vi "Oscilloscope.vi"(6 "Slow Control User":string, 9 "notifier in":T4, 10 "queue in":T3) -> ()   [LabVIEW 2012]
uses:
  TypeDefs/QueueNotifier/Notifier.ctl
  TypeDefs/QueueNotifier/DataQueue.ctl
  TypeDefs/DataTypes/SystemStatus.ctl
  TypeDefs/DataTypes/StopCondition.ctl
  TypeDefs/DataTypes/AcquisitionInfo.ctl
  TypeDefs/DataTypes/OscilloscopeState.ctl
  <vilib>/Analysis/6fits.llb/Remove Outliers (Range).vi
  <vilib>/Analysis/NI_AALPro.lvlib
panel:
  in  "Acquisition Info":T1 {"Shaping Amplifier" items=["CR-200-1us", "CR-200-100ns", "", ""]; "Preamplifier" items=["CR-Z-113-1k", "CR-Z-113-5k", "CR-Z-SiPM", ""]}
  out "Acquisition Rate":dbl format="%#.1f"
  in  "Stop":bool
  in  "Trigger Level (V)":dbl=-0.02
  in  "Range (V)":dbl(ring)=2.0 items=["10"=10.0, "5"=5.0, "2"=2.0, "1"=1.0, "0.4"=0.4, "0.2"=0.2, "0.08"=0.08, "0.04"=0.04, "0.02"=0.02, "0.01"=0.01]
  in  "Offset (V)":dbl=-0.5
  out "Acquiring Now?":bool
  out "Active Run?":bool
  out "Time Elapsed (s)":dbl format="%#.1f"
  out "Waveforms Acquired":dbl
  in  "Stop Condition":T2={"Quota"=2000.0, "Duration (S)"=120, "Stop Condition"=FALSE}
  in  "Run Info":bool caption="Configure DAQ"
  out "Signal":waveform(dbl)(graph)
  in  "Measurement (Ch1)":i32(ring)=26 items=["AC RMS"=1, "Amplitude"=2, "Average"=3, "Cycle Average"=4, "Cycle Frequency"=5, "Cycle Period"=6, "Cycle RMS"=7, "DC RMS"=8, "Estimated Number of Bits"=9, "Falling Edges"=10, "Fall Overshoot"=11, "Fall Preshoot"=12, "Frequency"=13, "Fall Crossing Time"=14, "Fall Time"=15, "High"=16, "Low"=17, "Maximum"=18, "Minimum"=19, "Mid"=20, "Negative Duty"=21, "Negative Width"=22, "Positive Duty"=23, "Period"=24, "Phase"=25, "Peak to Peak"=26, "Positive Width"=27, "Rising Edges"=28, "Rise Overshoot"=29, "Rise Preshoot"=30, "Rise Crossing Time"=31, "Rise Time"=32, "Standard Deviation"=33, "Spurious Free Dynamic Range"=34, "Signal to Noise+Distortion"=35, "Signal to Noise"=36, "Total Harmonic Distortion"=37, "Time of Maximum"=38, "Time of Minimum"=39]
  in  "New Run":bool caption="Configure DAQ"
  in  "Settings":bool caption="Configure DAQ"
  in  "Acquire":bool
  out "Preliminary Histogram":cluster{"Y":dbl[], "Y":dbl[]}[](graph)
  # "Shaper Gain"
  # "Self"
  # "Fast"
  # "Solicited"
  # "Standard"
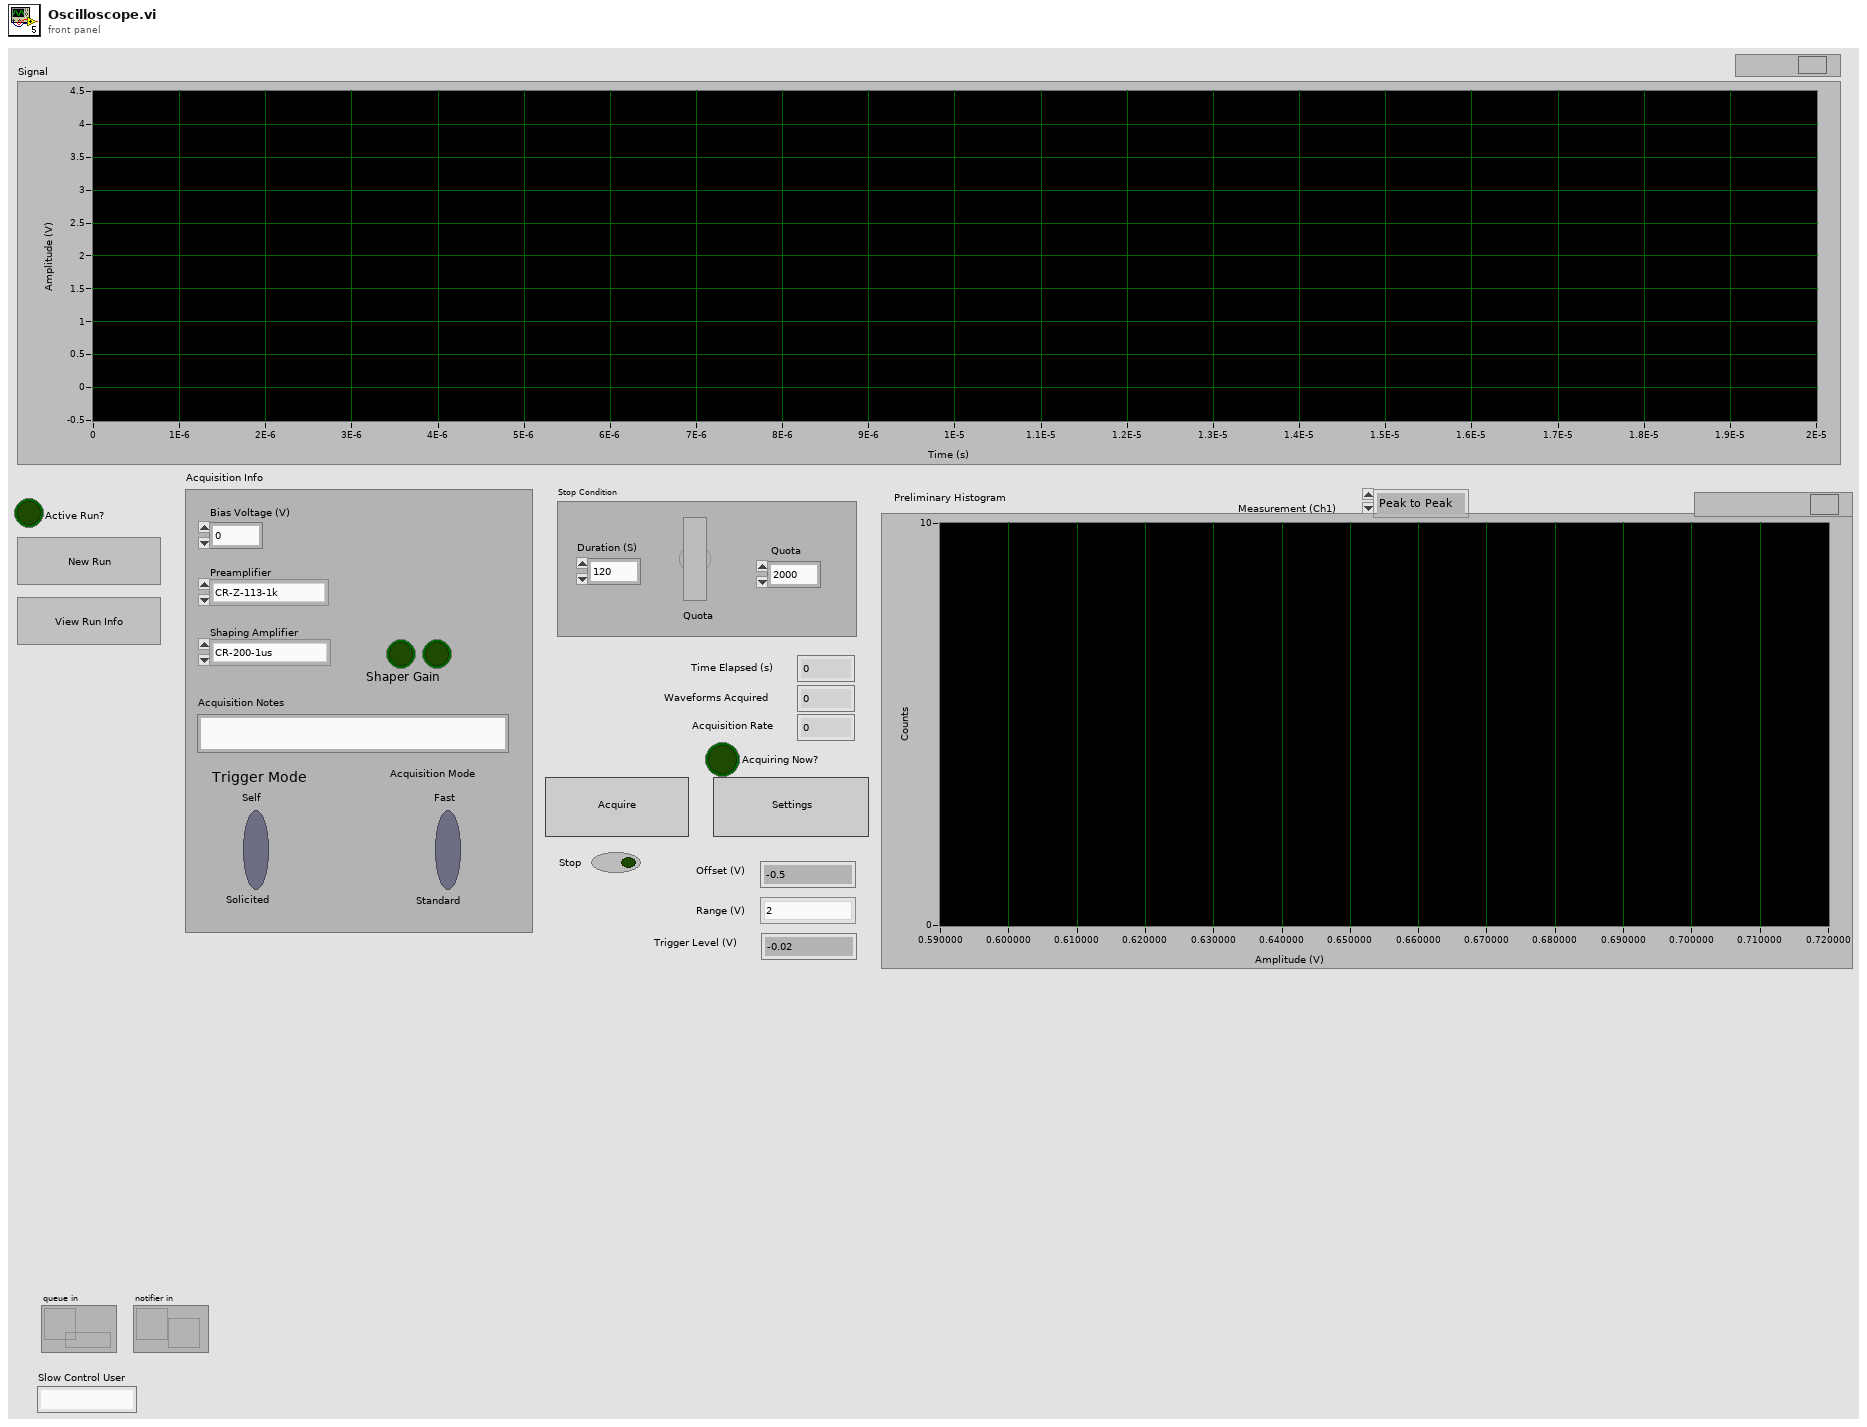
[diagram p1: front panel]
types:
  T1 = typedef "AcquisitionInfo.ctl" = cluster{"Trigger Mode":bool, "Acquisition Mode":bool, "Bias Voltage (V)":dbl, "Preamplifier":u16, "Shaping Amplifier":u16, "Acquisition Notes":string, "1":bool, "2":bool}
  T2 = typedef "StopCondition.ctl" = cluster{"Quota":dbl, "Duration (S)":u16, "Stop Condition":bool}
  T3 = typedef "DataQueue.ctl" = refnum<queue>
  T4 = typedef "Notifier.ctl" = refnum<notifier>
  T5 = typedef "OscilloscopeState.ctl" = enum16{"Acquire", "Initialize", "Waiting For Event", "New Run", "Settings", "Update UI", "ViewRunInfo", "Synchronize", "Fast Acquire"}
  T6 = typedef "Data.ctl" = cluster{"DAQ Config Data":T7, "Acquisition":T8, "Measurement":T10, "UI References":T11, "Run Info":T12, "System Status":T13, "Acquisition Info":cluster{"Trigger Mode":bool, "Acquisition Mode":bool, "Bias Voltage (V)":dbl, "Preamplifier":u16, "Shaping Amplifier":u16, "Acquisition Notes":string, "1":bool, "2":bool}}
  T7 = typedef "DAQConfig.ctl" = cluster{"Vertical":cluster{"Coupling":i32, "Offset (V)":dbl, "Range (V)":dbl, "Impedance":dbl}, "Horizontal":cluster{"Offset Time":dbl, "Sample Time (S)":dbl, "Sample Points":u32}, "Trigger\n":cluster{"Lower Level (V)":dbl, "Trigger Slope":i32, "Trigger Source":i32}, "Acquisition":cluster{"Trigger Mode":i32, "Initiate Continuously":i32, "Acquire Type":i32, "Acquire Count":i32}, "Channel":i32, "Instrument Handle":i32, "Error":errorcluster, "State":i32}
  T8 = typedef "Acquisition.ctl" = cluster{"Current":T9, "Stop Condition":T2, "Config Needed":bool}
  T9 = typedef "Current.ctl" = cluster{"Acquiring Now?":bool, "Waveforms Acquired":dbl, "Start of Acquisition":timestamp, "Acquisition Name":string}
  T10 = typedef "Measurement.ctl" = cluster{"Waveform":waveform(dbl), "Peak Heights":dbl[], "Acquisition Time":timestamp, "File Path":path, "TDMS File Handle":refnum<k34>}
  T11 = typedef "UIReferences.ctl" = cluster{"Acquire":refnum<vi>, "Configure DAQ":refnum<vi>, "Measurement (Ch1)":refnum<vi>, "Update Needed?":bool, "New Run":refnum<vi>, "Signal":refnum<vi>}
  T12 = typedef "RunInfo.ctl" = cluster{"Active Run?":bool, "Run Notes":string, "User Name":string, "Campaign ID#":string, "Run Name":string, "Start Time":timestamp, "End Time":timestamp}
  T13 = typedef "SystemStatus.ctl" = cluster{"Bias Voltage":dbl, "SiPM Temperature":dbl[], "Slow Control User":string, "LXe":dbl}
  T14 = enum8{"Enabled", "Disabled", "Disabled and Grayed Out"}
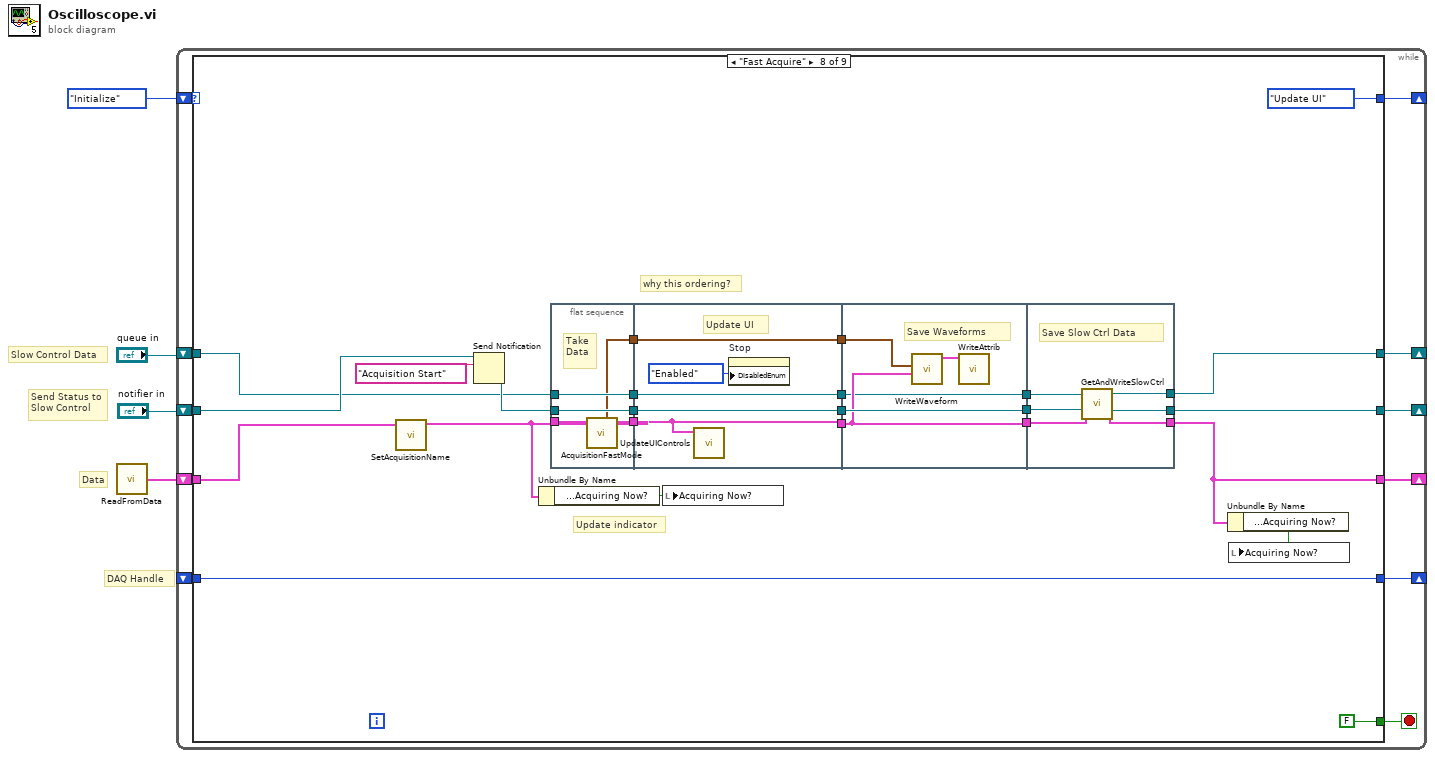
[diagram p0: block diagram]
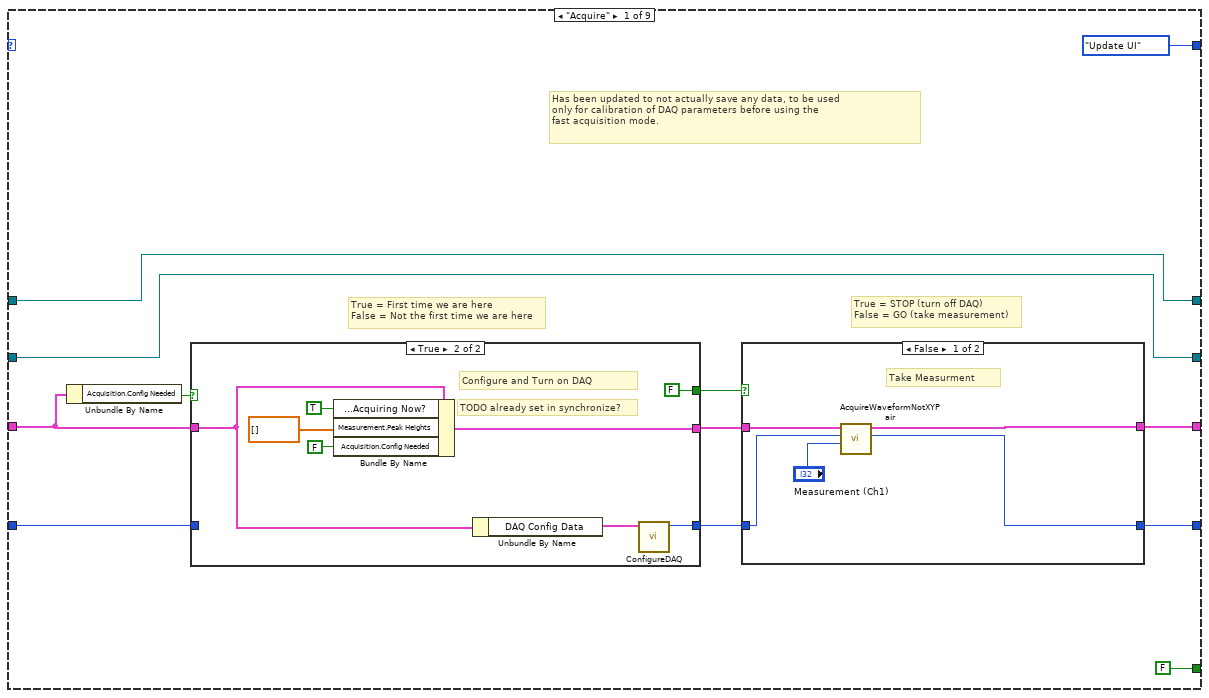
[diagram p2: hidden frame]
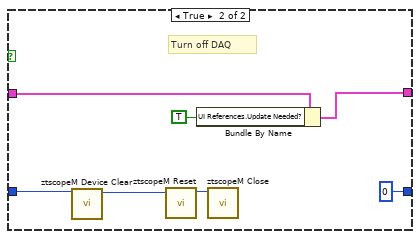
[diagram p3: hidden frame]
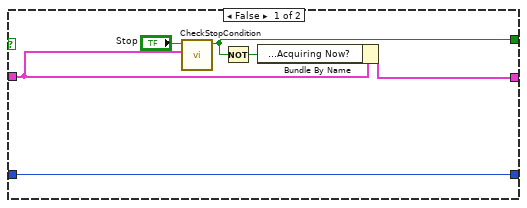
[diagram p4: hidden frame]
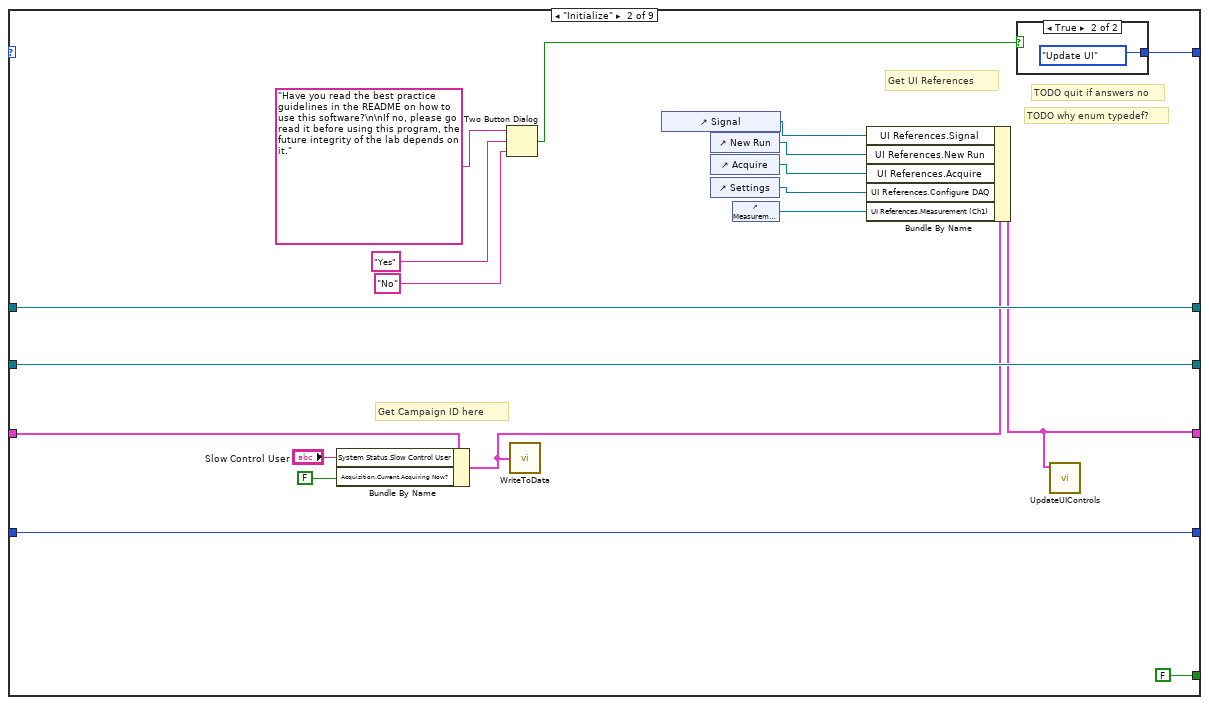
[diagram p5: hidden frame]
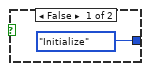
[diagram p6: hidden frame]
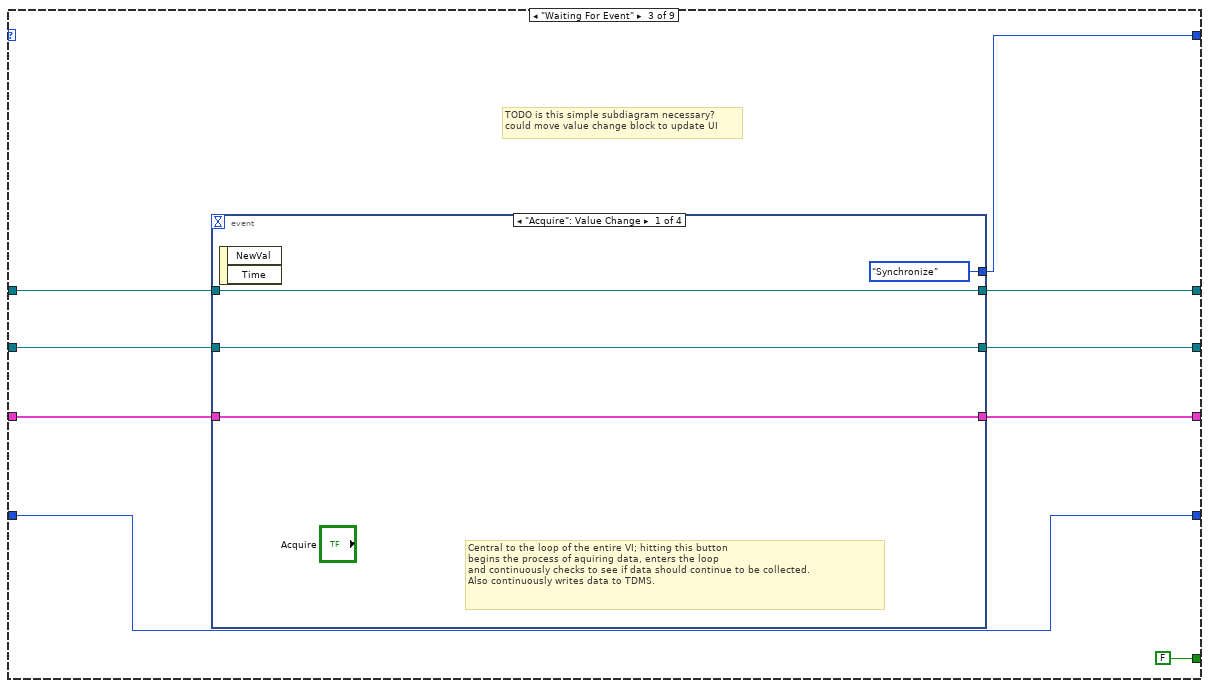
[diagram p7: hidden frame]
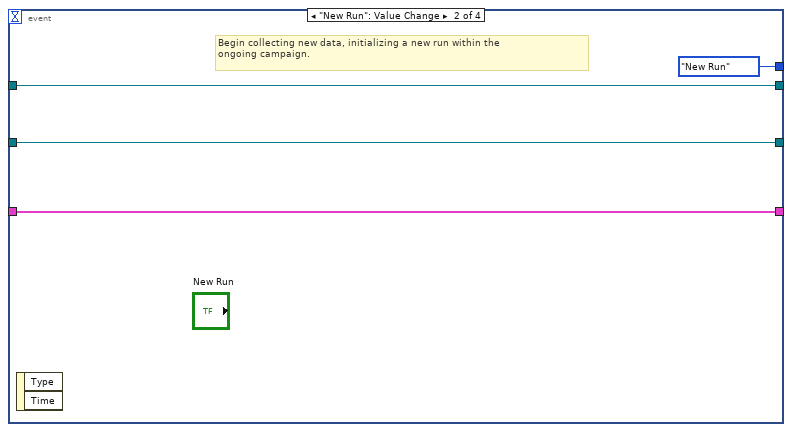
[diagram p8: hidden frame]
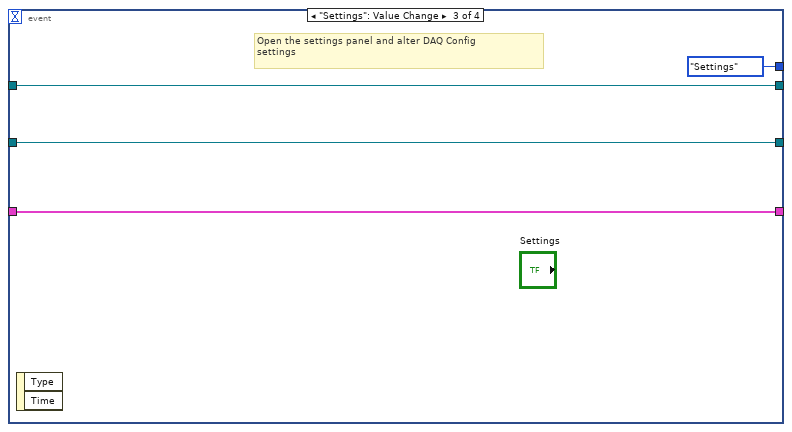
[diagram p9: hidden frame]
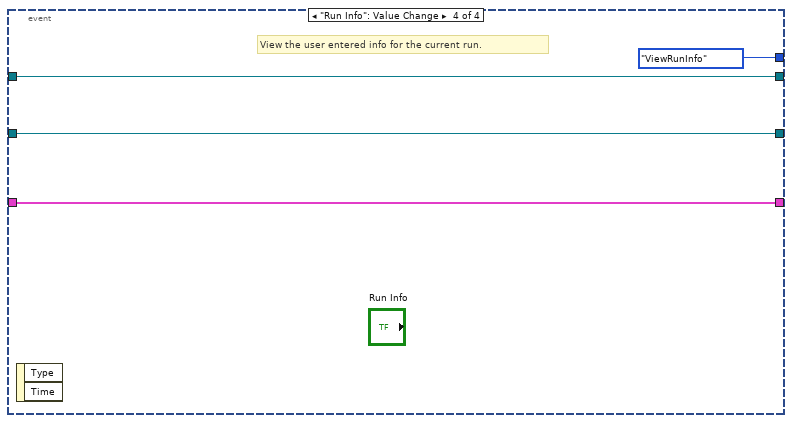
[diagram p10: hidden frame]
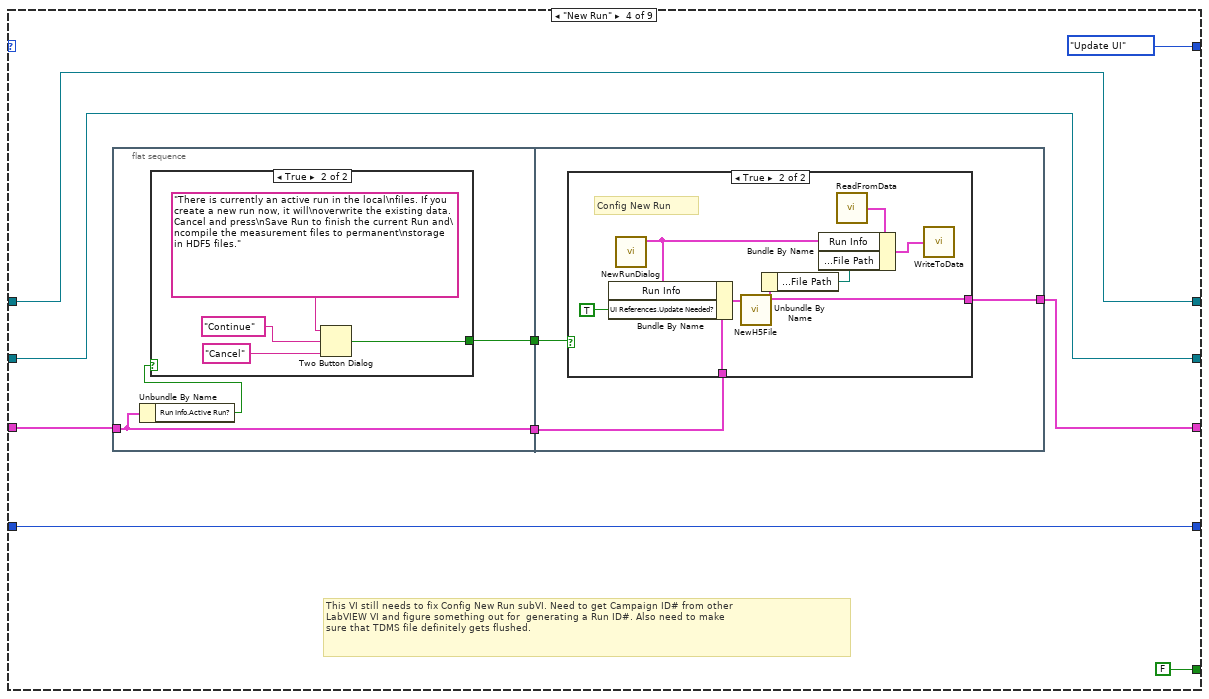
[diagram p11: hidden frame]
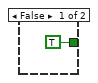
[diagram p12: hidden frame]
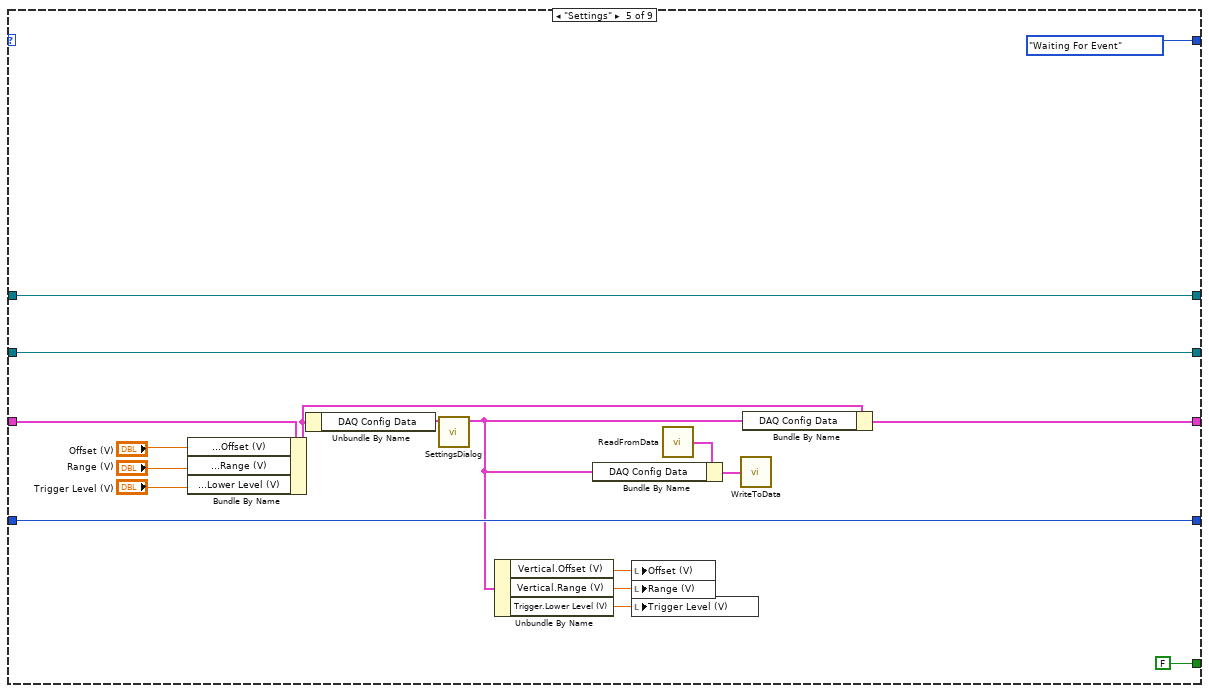
[diagram p14: hidden frame]
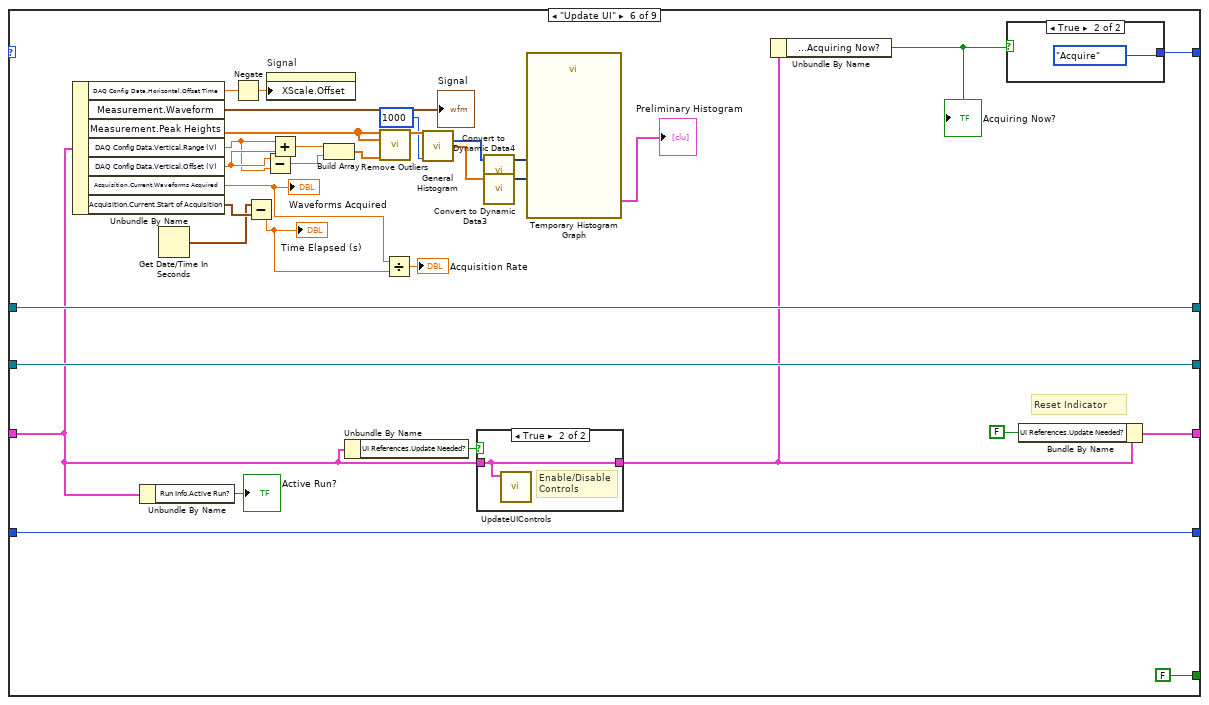
[diagram p15: hidden frame]
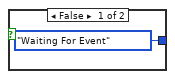
[diagram p16: hidden frame]
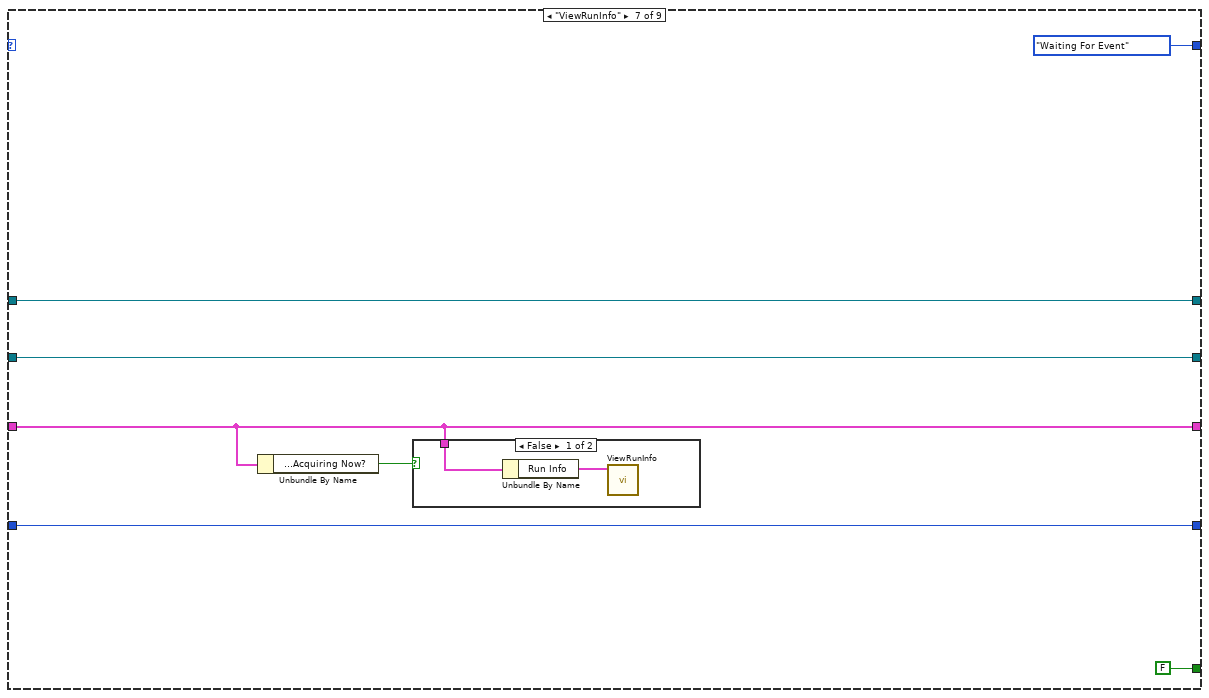
[diagram p18: hidden frame]
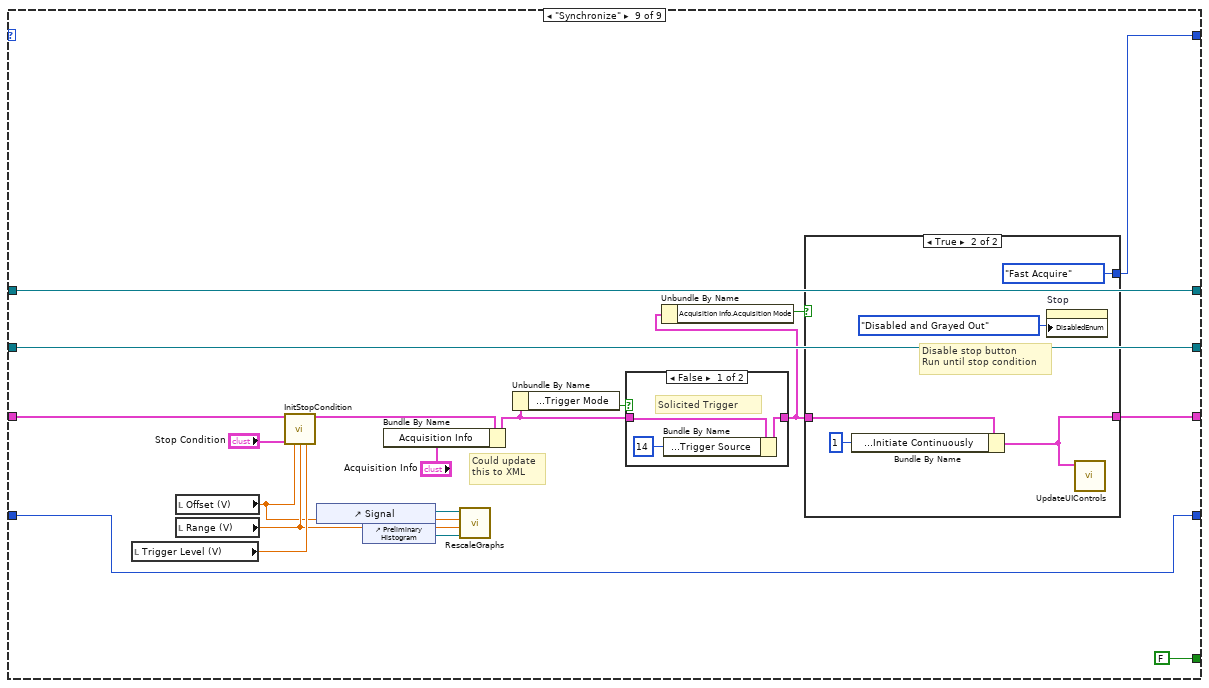
[diagram p20: hidden frame]
diagram:
  # "Data"
  # "Send Status to\nSlow Control"
  # "Slow Control Data"
  # "DAQ Handle"
  n1 = call "ReadFromData.vi"() -> ("Data"=w1:T6)  [unwired: 8 in]
  n2 = while {
    shift-right: [w14] -> _
    shift-left: _ -> [w15]
    shift-right: [w11] -> _
    shift-left: w1 -> [w13]
    shift-right: [w9] -> _
    shift-left: OscilloscopeState."Initialize" ("Enum") -> [w12]
    shift-right: [w8] -> _
    shift-left: "notifier in" -> [w5]
    shift-right: [w7] -> _
    shift-left: "queue in" -> [w6]
    stop <- w10 stop-if-true
    n3 = case shown="\"Fast Acquire\"" w12 {
      tunnel: [w24 w71 w82 w108 w142 w171 w188 w217 w241] -> w14
      tunnel: w15 -> [w21 w71 w82 w108 w142 w171 w188 w217 w241]
      tunnel: w13 -> [w19 w58 w75 w105 w133 w147 w185 w203 w240]
      tunnel: [OscilloscopeState."Update UI" ("Enum") w72 w76 OscilloscopeState."Update UI" ("Enum") OscilloscopeState."Waiting For Event" ("Enum") w175 OscilloscopeState."Waiting For Event" ("Enum") OscilloscopeState."Update UI" ("Enum") w251] -> w9
      tunnel: [w16 w55 w83 w103 w143 w172 w185 w205 w252] -> w11
      tunnel: [FALSE FALSE FALSE FALSE FALSE FALSE FALSE FALSE FALSE] -> w10
      tunnel: [w18 w60 w80 w100 w138 w167 w189 w204 w253] -> w8
      tunnel: w6 -> [w17 w61 w79 w101 w139 w168 w190 w207 w254]
      tunnel: [w17 w61 w78 w101 w139 w168 w190 w198 w254] -> w7
      tunnel: w5 -> [w18 w60 w77 w100 w138 w167 w189 w213 w253]
      frame "Acquire" {
        # "Has been updated to not actually save any data, to be used\nonly for calibration of DAQ parameters before using the\nfast acquisition mode."
        # "True = First time we are here\nFalse = Not the first time we are here"
        # "True = STOP (turn off DAQ)\nFalse = GO (take measurement)"
        n4 = Unbundle By Name(w19) -> ("Acquisition.Config Needed"=w27:bool)
        n5 = case shown="True" w27 {
          tunnel: w19 -> [w40 w50]
          tunnel: [w45 w47] -> w23
          tunnel: [w42 FALSE] -> w25
          tunnel: [w43 w52] -> w22
          tunnel: w21 -> [w43 _]
          frame False {
            n6 = call "CheckStopCondition.vi"("Data"=w40, "Stop"="Stop") -> ("f"=w42:bool)  [unwired: 9 in]
            n7 = Not(x=w42) -> (.not. x?=w44:bool)
            n8 = Bundle By Name(cluster=w40, "Acquisition.Current.Acquiring Now?"=w44) -> (w45:T6)
          }
          frame True {
            # "TODO already set in synchronize?"
            # "Configure and Turn on DAQ"
            n9 = Bundle By Name(cluster=w50, "Acquisition.Current.Acquiring Now?"=TRUE, "Measurement.Peak Heights"=dbl[] [], "Acquisition.Config Needed"=FALSE ("Acquisition.Current.Acquiring Now?")) -> (w47:T6)
            n10 = Unbundle By Name(w50) -> ("DAQ Config Data"=w51:T7)
            n11 = call "ConfigureDAQ.vi"("DAQ Config Data"=w51) -> ("Instrument Handle Out"=w52:i32)  [unwired: 9 in, 1 out]
          }
        }
        n12 = case shown="False" w25 {
          tunnel: w22 -> [w32 w38]
          tunnel: [w31 0 ("Instrument Handle Out out")] -> w24
          tunnel: w23 -> [w29 w33]
          tunnel: [w28 w35] -> w16
          frame False {
            # "Take Measurment"
            n13 = call "AcquireWaveformNotXYPair.vi"("Measurement (Ch1)"="Measurement (Ch1)", "Instrument Handle In"=w32, "Data in"=w29) -> ("Instrument Handle Out"=w31:i32, "Data out"=w28:T6)  [unwired: 6 in, 1 out]
          }
          frame True {
            # "Turn off DAQ"
            n14 = call <instrlib>:"ztscopeM Device Clear.vi"("Instrument Handle In"=w38) -> ("Instrument Handle Out"=w39:i32)  [unwired: 9 in, 1 out]
            n15 = call <instrlib>:"ztscopeM Reset.vi"("Instrument Handle In"=w39) -> ("Instrument Handle Out"=w37:i32)  [unwired: 9 in, 1 out]
            n16 = Bundle By Name(cluster=w33, "UI References.Update Needed?"=TRUE) -> (w35:T6)
            n17 = call <instrlib>:"ztscopeM Close.vi"("Instrument Handle In"=w37) -> ()  [unwired: 10 in, 1 out]
          }
        }
      }
      frame "Initialize" {
        # "TODO why enum typedef?"
        # "TODO quit if answers no"
        # "Get Campaign ID here"
        # "Get UI References"
        n18 = Bundle By Name(cluster=w58, "System Status.Slow Control User"="Slow Control User", "Acquisition.Current.Acquiring Now?"=FALSE) -> (w56:T6)
        n19 = Two Button Dialog(message="Have you read the best practice guidelines in the README on how to use this software?\n\nIf no, please go read it before using this program, the future integrity of the lab depends on it.", 1:"No" ("F button name (\"Cancel\")"), 2:"Yes" ("T button name (\"OK\")")) -> (T button?=w65:bool)
        n20 = call "WriteToData.vi"("Data"=w56) -> ()  [unwired: 6 in]
        n21 = control-ref of="Signal"() -> (w59:refnum<vi>)
        n22 = control-ref of="New Run"() -> (w64:refnum<vi>)
        n23 = control-ref of="Acquire"() -> (w63:refnum<vi>)
        n24 = control-ref of="Settings"() -> (w62:refnum<vi>)
        n25 = control-ref of="Measurement (Ch1)"() -> (w70:refnum<vi>)
        n26 = Bundle By Name(cluster=w56, "UI References.Signal"=w59, "UI References.New Run"=w64, "UI References.Acquire"=w63, "UI References.Configure DAQ"=w62, "UI References.Measurement (Ch1)"=w70) -> (w55:T6)
        n27 = case shown="True" w65 {
          tunnel: [OscilloscopeState."Initialize" ("Enum") OscilloscopeState."Update UI" ("Enum")] -> w72
          frame False {
          }
          frame True {
          }
        }
        n28 = call "UpdateUIControls.vi"("Data"=w55) -> ()  [unwired: 11 in]
      }
      frame "Waiting For Event" {
        # "TODO is this simple subdiagram necessary?\ncould move value change block to update UI"
        n29 = event shown="[0] \"Acquire\": Value Change" {
          selector: _ -> [_ _ _ _]
          dyn-events: _ -> [_ _ _ _]
          timeout: _ -> [_ _ _ _]
          tunnel: [OscilloscopeState."Synchronize" ("Enum") OscilloscopeState."New Run" ("Enum") OscilloscopeState."Settings" ("Enum") OscilloscopeState."ViewRunInfo" ("Enum")] -> w76
          tunnel: w75 -> [w86 w88 w92 w96]
          tunnel: [w86 w88 w92 w96] -> w83
          tunnel: w77 -> [w85 w89 w93 w97]
          tunnel: [w85 w89 w93 w97] -> w80
          tunnel: [w84 w90 w94 w98] -> w78
          tunnel: w79 -> [w84 w90 w94 w98]
          event "Acquire": Value Change {
            # "Central to the loop of the entire VI; hitting this button\nbegins the process of aquiring data, enters the loop \nand continuously checks to see if data should continue to be collected. \nAlso continuously writes data to TDMS."
            n30 = event-data() -> ()  [unwired: 1 in, 2 out]
          }
          event "New Run": Value Change {
            # "Begin collecting new data, initializing a new run within the \nongoing campaign."
            n31 = event-data() -> ()  [unwired: 1 in, 2 out]
          }
          event "Settings": Value Change {
            # "Open the settings panel and alter DAQ Config\nsettings"
            n32 = event-data() -> ()  [unwired: 1 in, 2 out]
          }
          event "Run Info": Value Change {
            # "View the user entered info for the current run."
            n33 = event-data() -> ()  [unwired: 1 in, 2 out]
          }
        }
      }
      frame "New Run" {
        # "This VI still needs to fix Config New Run subVI. Need to get Campaign ID# from other\nLabVIEW VI and figure something out for  generating a Run ID#. Also need to make\nsure that TDMS file definitely gets flushed."
        n34 = flat-sequence {
          tunnel: [w110] -> w106
          tunnel: w105 -> [w109]
          tunnel: [w109] -> w104
          tunnel: w106 -> [w119]
          tunnel: w104 -> [w118]
          tunnel: [w117] -> w103
          frame #0 {
            n35 = Unbundle By Name(w109) -> ("Run Info.Active Run?"=w111:bool)
            n36 = case shown="True" w111 {
              tunnel: [TRUE ("T button?") w115] -> w110
              frame False {
              }
              frame True {
                n37 = Two Button Dialog(message="There is currently an active run in the local\nfiles. If you create a new run now, it will\noverwrite the existing data. Cancel and press\nSave Run to finish the current Run and\ncompile the measurement files to permanent\nstorage in HDF5 files.", 1:"Cancel" ("F button name (\"Cancel\")"), 2:"Continue" ("T button name (\"OK\")")) -> (T button?=w115:bool)
              }
            }
          }
          frame #1 {
            n38 = case shown="True" w119 {
              tunnel: w118 -> [w120 w125]
              tunnel: [w120 w121] -> w117
              frame False {
              }
              frame True {
                # "Config New Run"
                n39 = call "NewRunDialog.vi"() -> ("Run Info Out"=w124:T12)  [unwired: 10 in]
                n40 = Bundle By Name(cluster=w125, "Run Info"=w124, "UI References.Update Needed?"=TRUE) -> (w123:T6)
                n41 = call "NewH5File.vi"("Data In"=w123) -> ("Data Out"=w121:T6)  [unwired: 10 in]
                n42 = Unbundle By Name(w121) -> ("Measurement.File Path"=w122:path)
                n43 = call "ReadFromData.vi"() -> ("Data"=w128:T6)  [unwired: 8 in]
                n44 = Bundle By Name(cluster=w128, "Run Info"=w124, "Measurement.File Path"=w122) -> (w127:T6)
                n45 = call "WriteToData.vi"("Data"=w127) -> ()  [unwired: 6 in]
              }
            }
          }
        }
      }
      frame "Settings" {
        n46 = Bundle By Name(cluster=w133, "DAQ Config Data.Vertical.Offset (V)"="Offset (V)", "DAQ Config Data.Vertical.Range (V)"="Range (V)", "DAQ Config Data.Trigger.Lower Level (V)"="Trigger Level (V)") -> (w132:T6)
        n47 = Unbundle By Name(w132) -> ("DAQ Config Data"=w144:T7)
        n48 = call "SettingsDialog.vi"("DAQ Config In"=w144) -> ("DAQ Config Out"=w137:T7)  [unwired: 8 in]
        n49 = Unbundle By Name(w137) -> ("Vertical.Offset (V)"=w136:dbl, "Vertical.Range (V)"=w135:dbl, "Trigger.Lower Level (V)"=w134:dbl)
        n50 = local write "Offset (V)"(w136) -> ()
        n51 = local write "Range (V)"(w135) -> ()
        n52 = local write "Trigger Level (V)"(w134) -> ()
        n53 = call "ReadFromData.vi"() -> ("Data"=w146:T6)  [unwired: 8 in]
        n54 = Bundle By Name(cluster=w146, "DAQ Config Data"=w137) -> (w145:T6)
        n55 = call "WriteToData.vi"("Data"=w145) -> ()  [unwired: 6 in]
        n56 = Bundle By Name(cluster=w132, "DAQ Config Data"=w137) -> (w143:T6)
      }
      frame "Update UI" {
        # "Reset Indicator"
        n57 = Unbundle By Name(w147) -> ("DAQ Config Data.Horizontal.Offset Time"=w161:dbl, "Measurement.Waveform"=→"Signal":waveform(dbl), "Measurement.Peak Heights"=w149:dbl[], "DAQ Config Data.Vertical.Range (V)"=w152:dbl, "DAQ Config Data.Vertical.Offset (V)"=w153:dbl, "Acquisition.Current.Waveforms Acquired"=w157:dbl, "Acquisition.Current.Start of Acquisition"=w159:timestamp)
        "Waveforms Acquired" <- w157
        n58 = Unbundle By Name(w147) -> ("Run Info.Active Run?"=→"Active Run?":bool)
        n59 = Get Date/Time In Seconds() -> (seconds since 1Jan1904=w158:timestamp)
        n60 = Negate(x=w161) -> (-x=w160:dbl)
        n61 = Subtract(x=w158, y=w159) -> (x-y=w164:dbl)
        "Time Elapsed (s)" <- w164
        n62 = Subtract(x=w153, y=w152) -> (x-y=w151:dbl)
        n63 = property on="Signal" class="WFGraph (strict)"("XScale.Offset"=w160) -> ()  [unwired: 2 in, 2 out]
        n64 = Add(x=w152, y=w153) -> (x+y=w154:dbl)
        n65 = Build Array(w154, w151) -> (w150:dbl[])
        n66 = Unbundle By Name(w147) -> ("UI References.Update Needed?"=w173:bool)
        n67 = call-poly <vilib>:"Remove Outliers.vi"("Y"=w149, "X"=w149, "Range"=w150) -> ("Y Out"=w155:dbl[])  [unwired: 8 in, 4 out]
        n68 = Divide(x=w157, y=w164) -> (x/y=→"Acquisition Rate":dbl)
        n69 = call <vilib>:"General Histogram.vi"("X"=w155, "# bins"=1000) -> ("Histogram"=w156:i32[], "Axis"=w178:dbl[])  [unwired: 9 in, 3 out]
        n70 = case shown="True" w173 {
          tunnel: w147 -> [w182 w183]
          tunnel: [w182 w183] -> w166
          frame False {
            # "Reduce \nOverhead"
          }
          frame True {
            # "Enable/Disable\nControls"
            n71 = call "UpdateUIControls.vi"("Data"=w183) -> ()  [unwired: 11 in]
          }
        }
        n72 = call "Convert to Dynamic Data4"("Array"=w156) -> ("Dynamic Data Type"=w176:dynamicdata)  [unwired: 3 in]
        n73 = call "Convert to Dynamic Data3"("Array"=w178) -> ("Dynamic Data Type"=w177:dynamicdata)  [unwired: 3 in]
        n74 = call "Temporary Histogram Graph"("Y Input"=w176, "X Input"=w177) -> ("XY Graph"=→"Preliminary Histogram":cluster{"Y":dbl[], "Y":dbl[]}[])  [unwired: 3 in, 6 out]
        n75 = Unbundle By Name(w166) -> ("Acquisition.Current.Acquiring Now?"=w169:bool)
        "Acquiring Now?" <- w169
        n76 = case shown="True" w169 {
          tunnel: [OscilloscopeState."Waiting For Event" ("Enum") OscilloscopeState."Acquire" ("Enum")] -> w175
          frame False {
          }
          frame True {
          }
        }
        n77 = Bundle By Name(cluster=w166, "UI References.Update Needed?"=FALSE) -> (w172:T6)
      }
      frame "ViewRunInfo" {
        n78 = Unbundle By Name(w185) -> ("Acquisition.Current.Acquiring Now?"=w184:bool)
        n79 = case shown="False" w184 {
          tunnel: w185 -> [w191 _]
          frame False {
            n80 = Unbundle By Name(w191) -> ("Run Info"=w192:T12)
            n81 = call "ViewRunInfo.vi"("Run Info In"=w192) -> ()  [unwired: 11 in]
          }
          frame True {
          }
        }
      }
      frame "Fast Acquire" {
        # "why this ordering?"
        # "Update indicator"
        n82 = call "SetAcquisitionName.vi"("Data In"=w203) -> ("Data Out"=w211:T6)  [unwired: 10 in]
        n83 = Send Notification(notification="Acquisition Start", notifier=w213) -> (notifier out=w209:T4)  [unwired: 1 in, 1 out]
        n84 = Unbundle By Name(w211) -> ("Acquisition.Current.Acquiring Now?"=w214:bool)
        n85 = flat-sequence {
          tunnel: w211 -> [w222]
          tunnel: [w221] -> w212
          tunnel: [w220] -> w210
          tunnel: w209 -> [w220]
          tunnel: [w219] -> w208
          tunnel: w207 -> [w219]
          tunnel: [w218] -> w206
          tunnel: w212 -> [w223]
          tunnel: w210 -> [w224]
          tunnel: w208 -> [w225]
          tunnel: w206 -> [w226]
          tunnel: [w226] -> w202
          tunnel: [w225] -> w201
          tunnel: [w224] -> w200
          tunnel: [w223] -> w199
          tunnel: w202 -> [w232]
          tunnel: w201 -> [w228]
          tunnel: w200 -> [w230]
          tunnel: w199 -> [w229]
          tunnel: [w229] -> w197
          tunnel: [w230] -> w196
          tunnel: [w228] -> w195
          tunnel: [w233] -> w204
          tunnel: [w235] -> w198
          tunnel: [w234] -> w205
          tunnel: w197 -> [w236]
          tunnel: w196 -> [w237]
          tunnel: w195 -> [w238]
          frame #0 {
            # "Take\nData"
            n86 = call "AcquisitionFastMode.vi"("Data In"=w222) -> ("Data Out"=w221:T6, "Waveforms"=w218:waveform(dbl)[])  [unwired: 8 in]
          }
          frame #1 {
            # "Update UI"
            n87 = call "UpdateUIControls.vi"("Data"=w223) -> ()  [unwired: 11 in]
            n88 = property on="Stop" class="Bool"("DisabledEnum"=T14."Enabled" ("Disabled")) -> ()  [unwired: 2 in, 2 out]
          }
          frame #2 {
            # "Save Waveforms"
            n89 = call "WriteWaveform.vi"("Data In"=w229, "Waveforms"=w232) -> ("Data Out"=w231:T6)  [unwired: 9 in]
            n90 = call "WriteAttrib.vi"("Data In"=w231) -> ()  [unwired: 11 in]
          }
          frame #3 {
            # "Save Slow Ctrl Data"
            n91 = call "GetAndWriteSlowCtrl.vi"("queue in"=w238, "notifier in"=w237, "Data In"=w236) -> ("queue out"=w235:T3, "notifier out"=w233:T4, "Data Out"=w234:T6)  [unwired: 5 in]
          }
        }
        n92 = local write "Acquiring Now?"(w214) -> ()
        n93 = Unbundle By Name(w205) -> ("Acquisition.Current.Acquiring Now?"=w194:bool)
        n94 = local write "Acquiring Now?"(w194) -> ()
      }
      frame "Synchronize" {
        # "Could update\nthis to XML"
        n95 = local read "Trigger Level (V)"() -> (w248:dbl)
        n96 = local read "Offset (V)"() -> (w243:dbl)
        n97 = local read "Range (V)"() -> (w244:dbl)
        n98 = call "InitStopCondition.vi"("Data"=w240, "Stop Condition"="Stop Condition", "Offset (V)"=w243, "Range (V)"=w244, "Trigger Level (V)"=w248) -> ("Data Out"=w247:T6)  [unwired: 10 in]
        n99 = control-ref of="Signal"() -> (w250:refnum<vi>)
        n100 = control-ref of="Preliminary Histogram"() -> (w249:refnum<vi>)
        n101 = Bundle By Name(cluster=w247, "Acquisition Info"="Acquisition Info") -> (w246:T6)
        n102 = call "RescaleGraphs.vi"("WaveformGraph in"=w250, "Offset (V) 3"=w243, "Range (V) 3"=w244, "Preliminary Histogram"=w249) -> ()  [unwired: 6 in]
        n103 = Unbundle By Name(w246) -> ("Acquisition Info.Trigger Mode"=w255:bool)
        n104 = case shown="False" w255 {
          tunnel: w246 -> [w258 w262]
          tunnel: [w259 w261] -> w245
          frame False {
            # "Solicited Trigger"
            n105 = Bundle By Name(cluster=w258, "DAQ Config Data.Trigger.Trigger Source"=14 ("DAQ Config Data.Trigger\n.Trigger Source")) -> (w259:T6)
          }
          frame True {
            # "Self Trigger"
            n106 = Bundle By Name(cluster=w262, "DAQ Config Data.Trigger.Trigger Source"=10 ("DAQ Config Data.Trigger\n.Trigger Source")) -> (w261:T6)
          }
        }
        n107 = Unbundle By Name(w245) -> ("Acquisition Info.Acquisition Mode"=w256:bool)
        n108 = case shown="True" w256 {
          tunnel: [OscilloscopeState."Acquire" ("t") OscilloscopeState."Fast Acquire" ("t")] -> w251
          tunnel: w245 -> [w268 w273]
          tunnel: [w264 w270] -> w252
          frame False {
            n109 = Bundle By Name(cluster=w268, "DAQ Config Data.Acquisition.Initiate Continuously"=0, "Acquisition.Config Needed"=TRUE ("UI References.Update Needed?"), "UI References.Update Needed?"=TRUE) -> (w264:T6)
          }
          frame True {
            # "Disable stop button\nRun until stop condition"
            n110 = Bundle By Name(cluster=w273, "DAQ Config Data.Acquisition.Initiate Continuously"=1) -> (w270:T6)
            n111 = property on="Stop" class="Bool"("DisabledEnum"=T14."Disabled and Grayed Out" ("Disabled")) -> ()  [unwired: 2 in, 2 out]
            n112 = call "UpdateUIControls.vi"("Data"=w270) -> ()  [unwired: 11 in]
          }
        }
      }
    }
  }
